vi "VI Permanent.vi"() -> ()   [LabVIEW 2020]
uses:
  Visualisierungs Elemente/Zahlen-Ausgabefeld.ctl
  Seiten/FT-IR/FGV FT-IR Aktionen.ctl
  Seiten/FT-IR/FGV FT-IR Diagnose Aktionen.ctl
  Allgemein/Ausgabefelder einfaerben Aktionen.ctl
  PNS/Aktionen FGV Istwerte.ctl
  Seiten/Anlagengrenzwerte/FGV Anlagengrenzwerte Aktionen.ctl
  cRIO/PC/Kommunikation mit cRIO.lvlib
  Seiten/FT-IR/FT-IR.lvlib
  Allgemein/allgemeine Sub-VIs.lvlib
  Stoerungen/Stoerungen.lvlib
  PNS/PNS.lvlib
  Seiten/Anlagengrenzwerte/Anlagengrenzwerte.lvlib
panel:
  out "Messgasverbrauc":T1 format="%.1f"
  out "Ist":T1 format="%.1f"
  out "Soll":T1 format="%.1f"
  out "Schaltschranktemp":T1 format="%.1f"
  out "Heizkreis FT-IR Messzelle":T1 format="%.1f"
  out "HL 1 PNS":T1 caption="Heizung Pumpe" format="%.1f"
  out "HL1":T1 caption="Heizleitung zu Filter" format="%.1f"
  out "Heizung Filter PNS":T1 caption="Heizung Filter" format="%.1f"
  out "Heizleitung zu FT-IR":T1 format="%.1f"
  out "Durchfluss FT-IR":T1 format="%.1f"
  out "Eingangsdruck FT-IR":T1 format="%.3f"
  out "Number of Scan":T1 format="%#_5g"
  out "aktive Störungen":string[](array[string])
  # "Allgemein"
  # "Messgasverbrauch Anlage"
  # "l/min"
  # "Messgasverbrauch Anlage"
  # "l/min"
  # "l/min"
  # "°C"
  # "Schaltschranktemperatur"
  # "Heizkreis FT-IR Messzelle"
  # "°C"
  # "Heizleitung 1 PNS"
  # "°C"
  # "Heizleitung zu PNS"
  # "°C"
  # "Heizung Filter PNS"
  # "°C"
  # "Heizleitung zu FT-IR"
  # "°C"
  # "Durchfluss FT-IR"
  # "l/min"
  # "Eingangsdruck FT-IR"
  # "atm"
  # "Number of Scan"
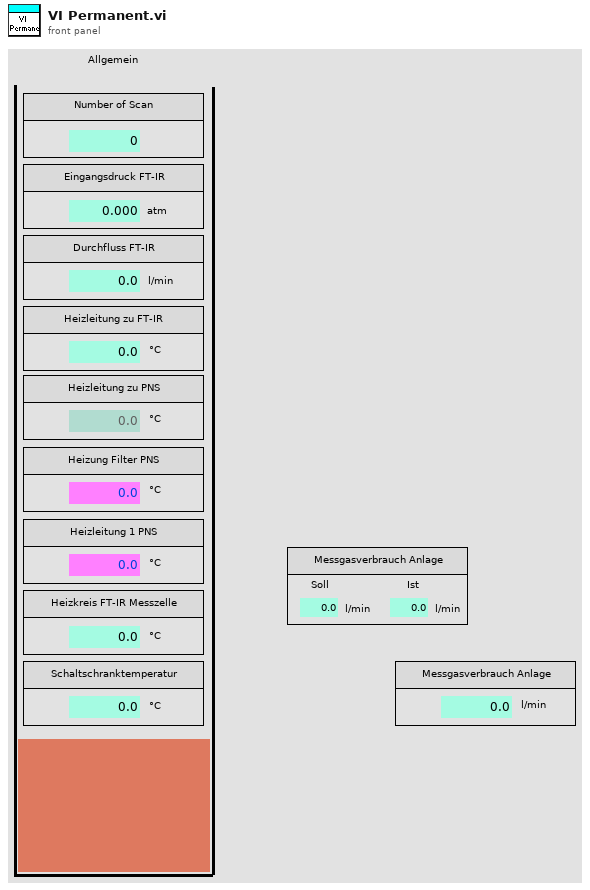
[diagram p1: front panel]
types:
  T1 = typedef "Zahlen-Ausgabefeld.ctl" = sgl
  T2 = typedef "PNS.lvlib/PNS Anlagenuebersicht.lvlib/PNS Ausgabefelder einfaerben Aktionen.ctl" = enum16{"lesen", "prüfen", "initialisieren"}
  T3 = typedef "allgemeine Sub-VIs.lvlib/Ausgabefelder einfaerben Aktionen.ctl" = enum16{"lesen", "prüfen", "initialisieren"}
  T4 = typedef "Anlagengrenzwerte.lvlib/FGV Anlagengrenzwerte Aktionen.ctl" = enum16{"Lesen", "Grenzwerte schreiben"}
  T5 = enum8{"Enabled", "Disabled", "Disabled and Grayed Out"}
  T6 = typedef "PNS.lvlib/Aktionen FGV Istwerte.ctl" = enum16{"lesen", "initialisieren", "schreiben", "Störungen"}
  T7 = typedef "FT-IR.lvlib/FGV FT-IR Diagnose Aktionen.ctl" = enum16{"Lesen", "Diagnose Schreiben", "Min Schreiben", "Max Schreiben"}
  T8 = typedef "FT-IR.lvlib/FGV FT-IR Aktionen.ctl" = enum16{"lesen", "NOG setzen", "NOS setzen", "Initialisieren", "speichern", "ALLES setzen", "FT-IR Spektrum loggen", "Komm Stoppen", "Spektrum LogKonfig"}
  T9 = typedef "Steuerung PNS.lvclass/Regler.ctl" = cluster{"Istwert":i16, "Sollwert":i16, "Alarm MIN":i16, "Alarm MAX":i16, "Regler sperren":i16, "Analog Ausgang":i16}[]
  T10 = typedef "Anlagengrenzwerte.lvlib/Anlagen-Grenzwerte Anzeige.ctl" = cluster{"Eingangsdruck FT-IR:":T11, "Durchfluss FT-IR:":T11, "Durchfluss CalGas:":T11, "Druck Ausgang:":T11, "Druck Kalter Block:":T11, "Heizleitungen intern:":T11, "Heizleitung zu FT-IR:":T11, "Heizung Filterblock:":T11, "Heizung Pumpe:":T11, "Heizleitung Extern SP1:":T11, "Heizleitung Extern SP2:":T11, "FT-IR Heizung Messzelle:":T11, "Schaltschranktemperatur:":T11, "Gaskühler:":T11}
  T11 = typedef "Anlagengrenzwerte.lvlib/Anlagen-Parameter Anzeige.ctl" = cluster{"Sollwert":sgl, "Warn-Min":sgl, "Warn-Max":sgl, "Abschalt-Min":sgl, "Abschalt-Max":sgl, "Regler":u16}
  T12 = cluster{"Istwert":i16, "Sollwert":i16, "Alarm MIN":i16, "Alarm MAX":i16, "Regler sperren":i16, "Analog Ausgang":i16}
  T13 = typedef "Verwaltung - cRIO.lvlib/Analog Eingaenge.ctl" = cluster{"AI0: Durchfluss FT-IR":sgl, "AI1: Druck Ausgang":sgl, "AI2: Umgebungsdruck":sgl, "AI3: Druck FT-IR":sgl, "AI4: Druck CalGas":sgl, "AI5: Reserve":sgl, "AI6: Reserve":sgl, "AI7: Reserve":sgl, "Rohwert Durchfluss FT-IR":sgl, "Rohwert Druck Ausgang":sgl, "Rohwert Umgebungsdruck":sgl, "Rohwert Druck FT-IR":sgl, "Rohwert Druck CalGas":sgl, "Rohwert AI5":sgl, "Rohwert AI6":sgl, "Rohwert AI7":sgl, "Rohwert Diffdruck mbar FTIR":sgl}
  T14 = typedef "Verwaltung - cRIO.lvlib/TC Eingaenge.ctl" = cluster{"TC0: Reserve":sgl, "TC1: HL zu FT-IR":sgl, "TC2: HL Extern SP1":sgl, "TC3: HL Extern SP2":sgl, "TC4: Reserve":sgl, "TC5: Reserve":sgl, "TC6: Reserve":sgl, "TC7: Reserve":sgl, "TC8: FT-IR":sgl, "TC9: Reserve":sgl, "TC10: Schaltschrank":sgl, "TC11: Umgebung":sgl}
  T15 = typedef "Zahlen-Eingabefeld.ctl" = sgl
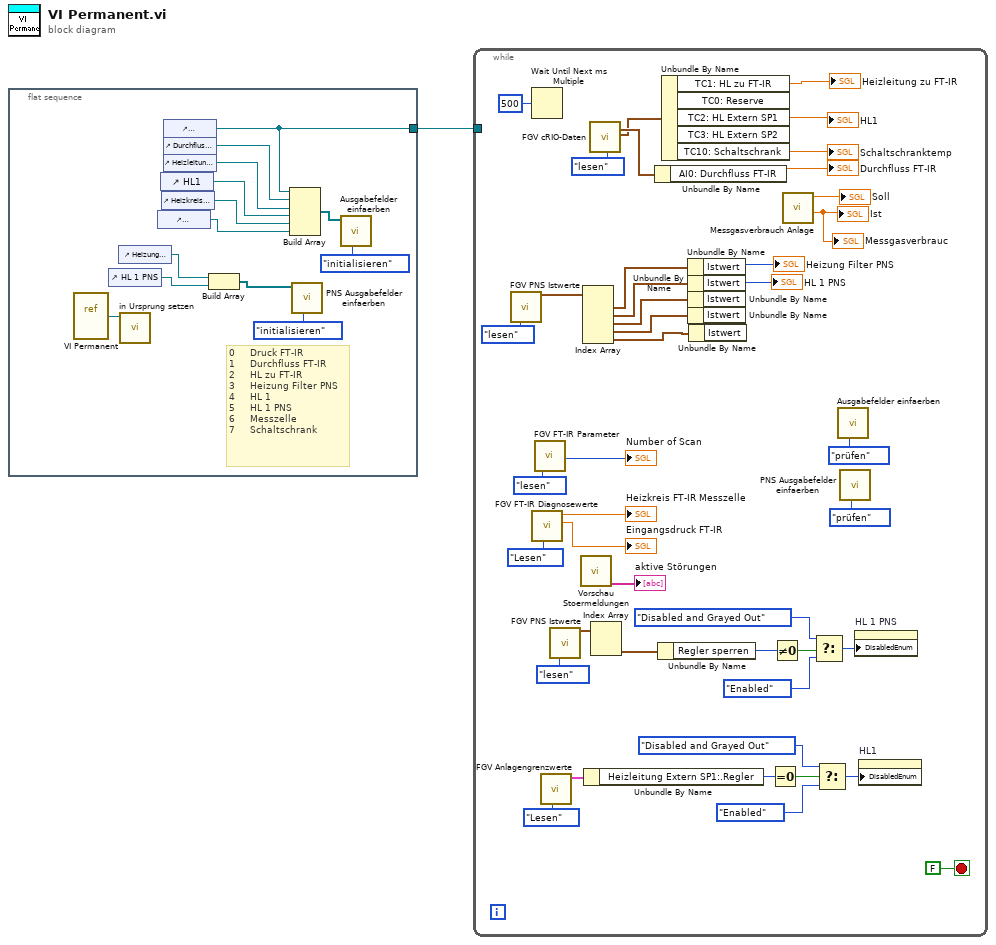
[diagram p0: block diagram]
diagram:
  n1 = flat-sequence {
    tunnel: [w9] -> w1
    frame #0 {
      # "0     Druck FT-IR\n1     Durchfluss FT-IR\n2     HL zu FT-IR\n3     Heizung Filter PNS\n4     HL 1\n5     HL 1 PNS\n6     Messzelle\n7     Schaltschrank"
      n2 = vi-ref "VI Permanent.vi"() -> (w10:refnum<vi>)
      n3 = control-ref of="HL 1 PNS"() -> (w3:refnum<vi>)
      n4 = control-ref of="Heizung Filter PNS"() -> (w4:refnum<vi>)
      n5 = call "in Ursprung setzen.vi"("VI Referenz"=w10) -> ()  [unwired: 10 in, 1 out]
      n6 = control-ref of="Schaltschranktemp"() -> (w6:refnum<vi>)
      n7 = control-ref of="HL1"() -> (w8:refnum<vi>)
      n8 = control-ref of="Heizkreis FT-IR Messzelle"() -> (w7:refnum<vi>)
      n9 = control-ref of="Eingangsdruck FT-IR"() -> (w9:refnum<vi>)
      n10 = control-ref of="Durchfluss FT-IR"() -> (w11:refnum<vi>)
      n11 = control-ref of="Heizleitung zu FT-IR"() -> (w12:refnum<vi>)
      n12 = Build Array(w4, w3) -> (w2:refnum<vi>[])
      n13 = Build Array(w9, w11, w12, w8, w7, w6) -> (w13:refnum<vi>[])
      n14 = call "PNS Ausgabefelder einfaerben.vi"("Aktionen"=PNS_Ausgabefelder_einfaerben_Aktionen."initialisieren", "Angehängtes Array"=w2) -> ()  [unwired: 10 in]
      n15 = call "Ausgabefelder einfaerben.vi"("Aktionen"=Ausgabefelder_einfaerben_Aktionen."initialisieren", "Angehängtes Array"=w13) -> ()  [unwired: 10 in]
    }
  }
  n16 = while {
    tunnel: w1 -> [_]
    stop <- FALSE stop-if-true
    n17 = call "FGV PNS Istwerte.vi"("Aktionen"=Aktionen_FGV_Istwerte."lesen") -> ("Regler"=w39:T9)  [unwired: 11 in, 3 out]
    n18 = Wait Until Next ms Multiple(millisecond multiple=u32 500 ("Vielfache von ms")) -> ()  [unwired: 1 out]
    n19 = call "FGV FT-IR Diagnosewerte.vi"("Aktionen"=FGV_FT-IR_Diagnose_Aktionen."Lesen") -> ("Druck"=→"Eingangsdruck FT-IR":dbl, "Temperatur"=→"Heizkreis FT-IR Messzelle":dbl)  [unwired: 5 in, 4 out]
    n20 = call "FGV FT-IR Parameter.vi"("Aktion"=FGV_FT-IR_Aktionen."lesen") -> ("NoOfScan"=→"Number of Scan":u32)  [unwired: 11 in, 7 out]
    n21 = call "FGV Anlagengrenzwerte.vi"("Aktion"=FGV_Anlagengrenzwerte_Aktionen."Lesen") -> ("Anlagen-Grenzwerte Anzeige"=w16:T10)  [unwired: 1 in, 9 out]
    n22 = call "FGV PNS Istwerte.vi"("Aktionen"=Aktionen_FGV_Istwerte."lesen") -> ("Regler"=w27:T9)  [unwired: 11 in, 3 out]
    n23 = call "Vorschau Stoermeldungen.vi"() -> ("Vorschau Störungen"=→"aktive Störungen":string[])  [unwired: 10 in, 1 out]
    n24 = Index Array(array=w39) -> (element #1=w34:T12, element #2=w38:T12, element #3=w37:T12, element #4=w36:T12, element #5=w33:T12)  [unwired: 5 in]
    n25 = Unbundle By Name(w16) -> ("Heizleitung Extern SP1:.Regler"=w15:u16)
    n26 = call "FGV cRIO-Daten.vi"("Aktion"=enum16{"lesen", "schreiben"}."lesen") -> ("Analog Input"=w49:T13, "TC Eingänge"=w45:T14)  [unwired: 9 in, 8 out]
    n27 = Index Array(array=w27) -> (element #2=w28:T12)  [unwired: 2 in, 1 out]
    n28 = Unbundle By Name(w49) -> ("AI0: Durchfluss FT-IR"=→"Durchfluss FT-IR":sgl)
    n29 = Unbundle By Name(w28) -> ("Regler sperren"=w29:i16)
    n30 = Unbundle By Name(w45) -> ("TC1: HL zu FT-IR"=→"Heizleitung zu FT-IR":sgl, "TC2: HL Extern SP1"=→"HL1":sgl, "TC10: Schaltschrank"=→"Schaltschranktemp":sgl)  [unwired: 2 out]
    n31 = Unbundle By Name(w34) -> ("Istwert"=→"Heizung Filter PNS":i16)
    n32 = Unbundle By Name(w38) -> ("Istwert"=→"HL 1 PNS":i16)
    n33 = Unbundle By Name(w37) -> ()  [unwired: 1 out]
    n34 = Unbundle By Name(w36) -> ()  [unwired: 1 out]
    n35 = Unbundle By Name(w33) -> ()  [unwired: 1 out]
    n36 = Equal To 0?(x=w15) -> (x = 0?=w21:bool)
    n37 = Not Equal To 0?(x=w29) -> (x != 0?=w26:bool)
    n38 = call "Messgasverbrauch Anlage.vi"() -> ("Ist-Flow"=→"Ist" →"Messgasverbrauc":sgl, "Soll-Flow"=→"Soll":T15)  [unwired: 10 in]
    n39 = Select(t=T5."Disabled and Grayed Out" ("Deaktiviert"), s=w26, f=T5."Enabled" ("Deaktiviert")) -> (s? t:f=w25:T5)
    n40 = Select(t=T5."Disabled and Grayed Out" ("Deaktiviert"), s=w21, f=T5."Enabled" ("Deaktiviert")) -> (s? t:f=w18:T5)
    n41 = call "Ausgabefelder einfaerben.vi"("Aktionen"=Ausgabefelder_einfaerben_Aktionen."prüfen") -> ()  [unwired: 11 in]
    n42 = call "PNS Ausgabefelder einfaerben.vi"("Aktionen"=PNS_Ausgabefelder_einfaerben_Aktionen."prüfen") -> ()  [unwired: 11 in]
    n43 = property on="HL 1 PNS" class="DigWert (strikt)"("DisabledEnum"=w25) -> ()  [unwired: 2 in, 2 out]
    n44 = property on="HL1" class="DigWert (strikt)"("DisabledEnum"=w18) -> ()  [unwired: 2 in, 2 out]
  }
